vi "Frame Array File Handler.vi"(7 "launch utility?":bool, 8 "error in":errorcluster, 10 "selected frame array file":path, 11 "configuration file page data":T1 {"custom device ref" format="%.0x"}) -> (0 "error out":errorcluster, 3 "configuration file page data out":T1 {"custom device ref" format="%.0x"})   [LabVIEW 2020, in "AIM ARINC 664 System Explorer.lvlib" / "Implementation.lvlib"]
uses:
  Implementation.lvlib
  Types/Configuration File Page Data.ctl
  Types/Path Control.ctl
  Types/Browse Button.ctl
  <vilib>/NI VeriStand/Custom Device API/Custom Device Item Ref.ctl
  Scripting/AIM ARINC 664 Scripting.lvlib
  Frame Configuration/FrameEditor.lvlib
  <vilib>/NI VeriStand/Custom Device API/Custom Device API.lvlib
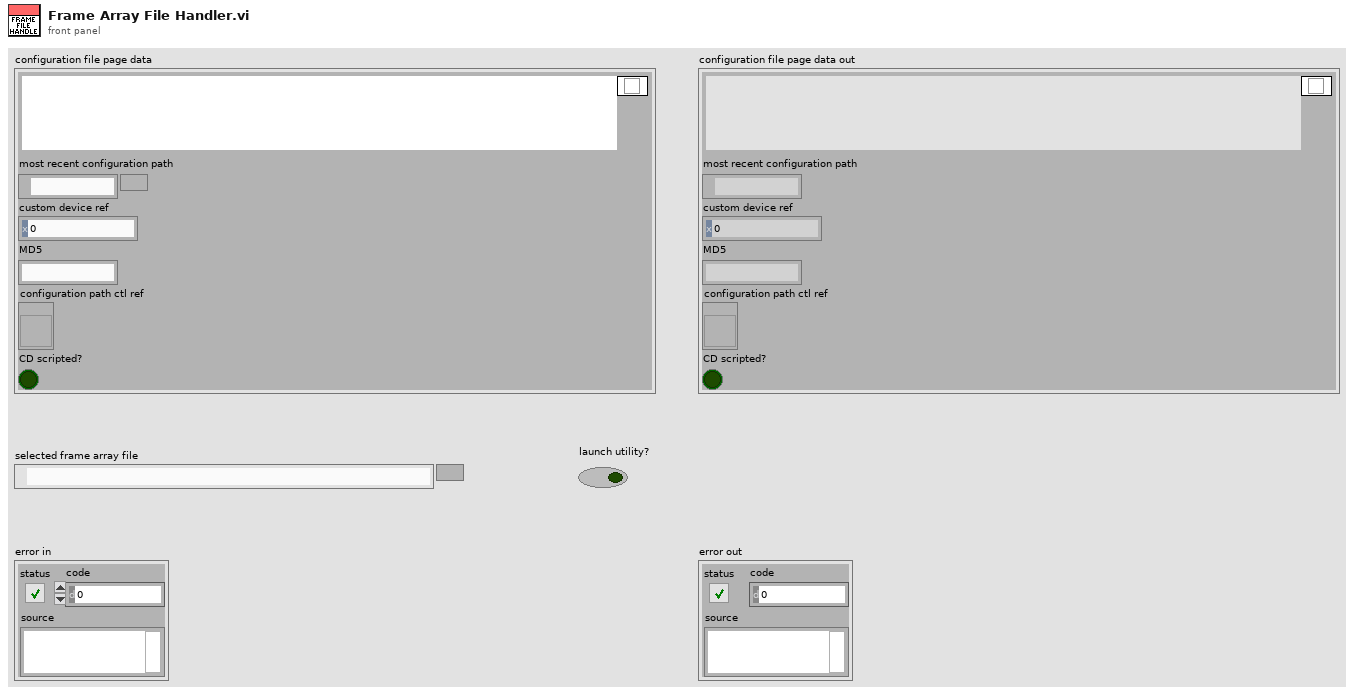
[diagram p1: front panel]
types:
  T1 = typedef "AIM ARINC 664 System Explorer.lvlib/Implementation.lvlib/Configuration File Page Data.ctl" = cluster{"Parameters":T2, "most recent configuration path":path, "custom device ref":T4, "MD5":string, "configuration path ctl ref":refnum<vi>, "CD scripted?":bool}
  T2 = typedef "AIM ARINC 664 System Explorer.lvlib/Implementation.lvlib/Path Control.ctl" = cluster{"file path":path, "Browse":T3}
  T3 = typedef "AIM ARINC 664 System Explorer.lvlib/Implementation.lvlib/Browse Button.ctl" = bool
  T4 = typedef "Custom Device API.lvlib/Custom Device Item Ref.ctl" = u64
  T5 = typedef "Payload Map.ctl" = map{string, T6}
  T6 = typedef "Payload Record Type.ctl" = cluster{"Data":u8[], "Type of Frame":T7}
  T7 = typedef "Type of Payload.ctl" = u16
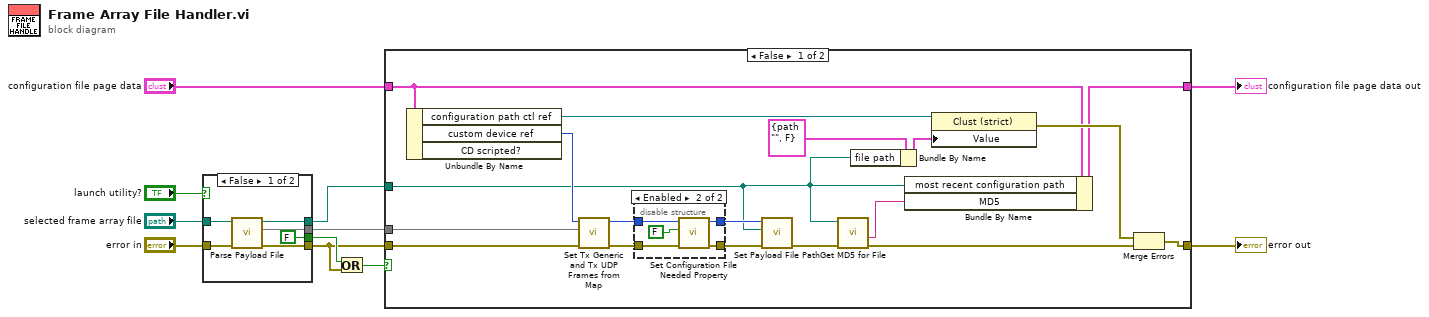
[diagram p0: block diagram]
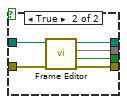
[diagram p2: hidden frame]
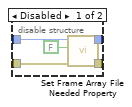
[diagram p3: hidden frame]
diagram:
  n1 = case shown="False" "launch utility?" {
    tunnel: "selected frame array file" -> [w17 w19]
    tunnel: [w16 w21] -> w7
    tunnel: [w15 w20] -> w6
    tunnel: "error in" -> [w14 w23]
    tunnel: [w13 w22] -> w1
    tunnel: [FALSE w18] -> w2
    frame False {
      n2 = call "Parse Payload File.vi"("error in"=w14, "frame array path in"=w17) -> ("error out"=w13:errorcluster, "Map"=w16:T5, "frame array path out"=w15:path)  [unwired: 7 in]
    }
    frame True {
      n3 = call "Frame Editor.vi"("error in"=w23, "Input File"=w19) -> ("error out"=w22:errorcluster, "Cancelled"=w18:bool, "Output Map"=w21:T5, "Currently Loaded file"=w20:path)  [unwired: 6 in]
    }
  }
  n4 = Or(x=w2, y=w1) -> (x .or. y?=w3:bool)
  n5 = case shown="False" w3 {
    tunnel: "configuration file page data" -> [w40 w53]
    tunnel: [w31 w53] -> w10
    tunnel: [w39 w52] -> w9
    tunnel: w7 -> [w26 _]
    tunnel: w6 -> [w25 _]
    tunnel: w1 -> [w24 w52]
    frame False {
      n6 = Unbundle By Name(w40) -> ("configuration path ctl ref"=w38:refnum<vi>, "custom device ref"=w32:T4)  [unwired: 1 out]
      n7 = call "Set Tx Generic and Tx UDP Frames from Map.vi"("error in"=w24, "payload map"=w26, "custom device ref"=w32) -> ("error out"=w37:errorcluster, "custom device ref out"=w33:T4)  [unwired: 7 in]
      n8 = disable-structure shown="Enabled" {
        disable-tunnel: w37 -> [w46 w50]
        disable-tunnel: w33 -> [w45 w48]
        disable-tunnel: [w43 w49] -> w30
        disable-tunnel: [w42 w47] -> w27
        frame Disabled {
          n9 = call "Set Frame Array File Needed Property.vi"("error in"=w46, "needed?"=FALSE, "custom device ref in"=w45) -> ("error out"=w43:errorcluster, "custom device ref out"=w42:T4)  [unwired: 7 in]
        }
        frame Enabled {
          n10 = call "Set Configuration File Needed Property.vi"("error in"=w50, "needed?"=FALSE, "custom device ref in"=w48) -> ("error out"=w49:errorcluster, "custom device ref out"=w47:T4)  [unwired: 7 in]
        }
      }
      n11 = call "Set Payload File Path.vi"("error in"=w30, "frame array file path"=w25, "custom device ref in"=w27) -> ("error out"=w28:errorcluster)  [unwired: 7 in, 1 out]
      n12 = call "Get MD5 for File.vi"("error in"=w28, "Path"=w25) -> ("error out"=w29:errorcluster, "MD5"=w36:string)  [unwired: 8 in]
      n13 = Bundle By Name(cluster=T2 {"file path"=path "", "Browse"=FALSE} ("Path"), "file path"=w25) -> (w34:T2)
      n14 = Bundle By Name(cluster=w40, "most recent configuration path"=w25, "MD5"=w36) -> (w31:T1)
      n15 = property class="Clust (strict)"(reference=w38, "Value"=w34) -> (error out=w41:errorcluster)  [unwired: 1 in, 1 out]
      n16 = Merge Errors(w41, w29) -> (w39:errorcluster)
    }
    frame True {
      # "Error or cancelled"
    }
  }
  "configuration file page data out" <- w10
  "error out" <- w9
